vi "SWLDA_Weight_Multiplier.vi"(8 "Z_array":dbl[][](array[numeric]), 11 "Weight":dbl[](array[numeric])) -> (3 "CSP Processed\nSWSVM Array":dbl[][](array[numeric]))   [LabVIEW 2014]
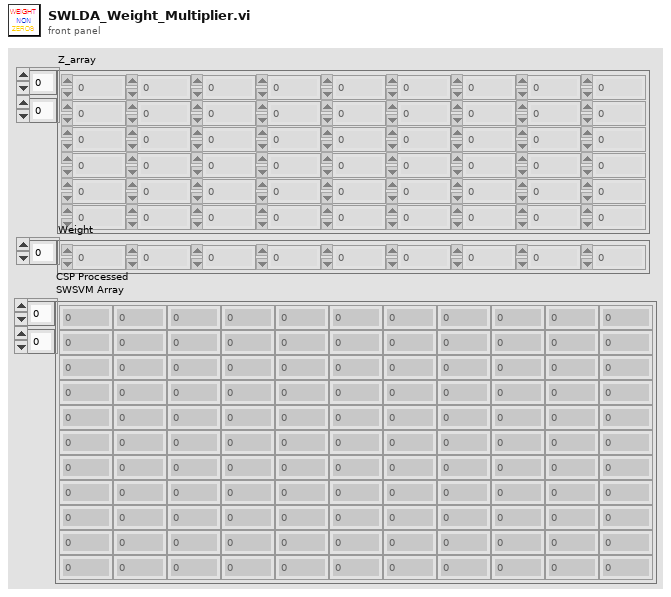
[diagram p1: front panel]
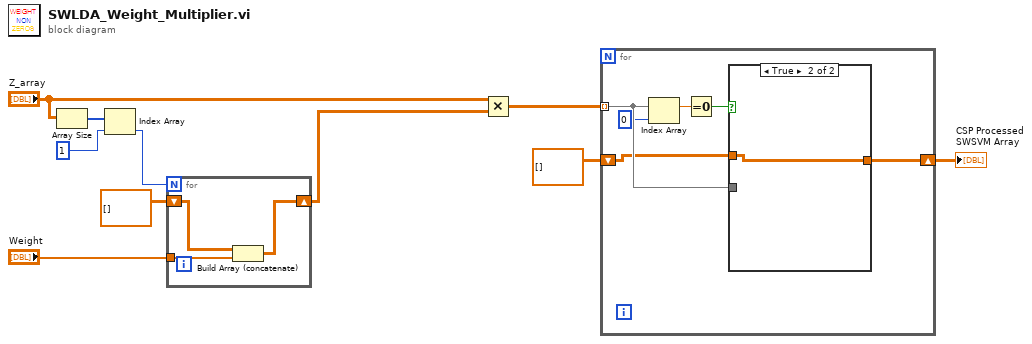
[diagram p0: block diagram]
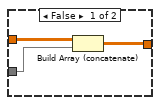
[diagram p2: hidden frame]
diagram:
  n1 = Array Size(array="Z_array") -> (size(s)=w4:i32[])
  n2 = Index Array(array=w4, index=1) -> (element=w2:i32)
  n3 = for {
    N: w2 -> [_]
    tunnel: "Weight" -> [w13]
    shift-right: [w12] -> w1
    shift-left: dbl[][] [] -> [w11]
    n4 = Build Array (concatenate)(w11, w13) -> (w12:dbl[][])
  }
  n5 = Multiply(x="Z_array", y=w1) -> (x*y=w10:dbl[][])
  n6 = for {
    tunnel: w10 -> [w19] mode=indexing
    shift-right: [w14] -> w8
    shift-left: dbl[][] [] -> [w18]
    n7 = Index Array(array=w19, index=0) -> (element=w17:dbl)
    n8 = Equal To 0?(x=w17) -> (x = 0?=w15:bool)
    n9 = case shown="True" w15 {
      tunnel: w19 -> [w22 _]
      tunnel: [w21 w23] -> w14
      tunnel: w18 -> [w20 w23]
      frame False {
        n10 = Build Array (concatenate)(w20, w22) -> (w21:dbl[][])
      }
      frame True {
      }
    }
  }
  "CSP Processed\nSWSVM Array" <- w8
